vi "Insert Subroutine.vi"(8 "error in (no error)":errorcluster, 10 "Insert Subroutine":T1, 11 "Test Executive Builder in":refnum<class "Test Executive Builder.lvclass">) -> (0 "error out":errorcluster, 3 "Test Executive Builder out":refnum<class "Test Executive Builder.lvclass">, 5 "Unique ID out":string)   [LabVIEW 2017, in "Test Executive Builder.lvclass"]
uses:
  Test Executive Builder.lvclass
  Source/Test Executive Builder Model/Test Executive Builder Model/Test Executive Builder Model.lvclass
  e5ad1a27-23be-4da1-be5e-5f15b9041f0f.vi
  <vilib>/gpm_packages/@cs/mva-core/Source/IModel/IModel/IModel.lvclass
  C:/Users/jonmc/Documents/Git/Test Executive Builder/Source/Test Executive Builder Model/Test Executive Builder Model/Test Executive Builder Model.lvclass
  C:/Users/jonmc/Documents/Git/Test Executive Builder/gpm_packages/@cs/mva-core/Source/IModel/IModel/IModel.lvclass
  Source/Test Executive Builder Dialogs/ITest Executive Builder Dialog/ITest Executive Builder Dialog.lvclass
  Source/Application Dependencies/Insert Subroutine.ctl
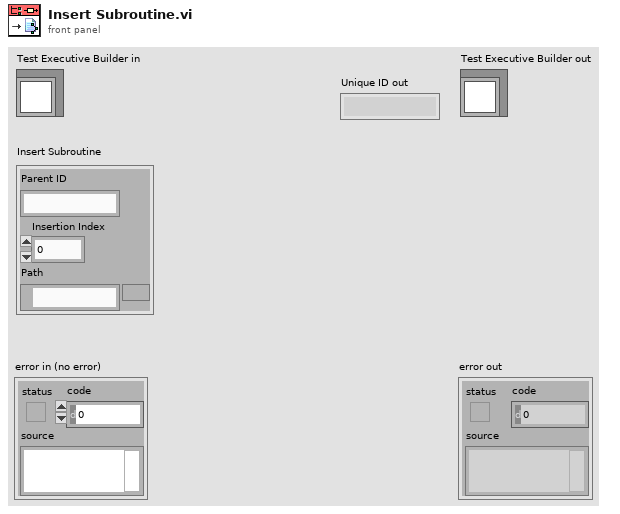
[diagram p1: front panel]
types:
  T1 = typedef "Insert Subroutine.ctl" = cluster{"Parent ID":string, "Insertion Index":i32, "Path":path}
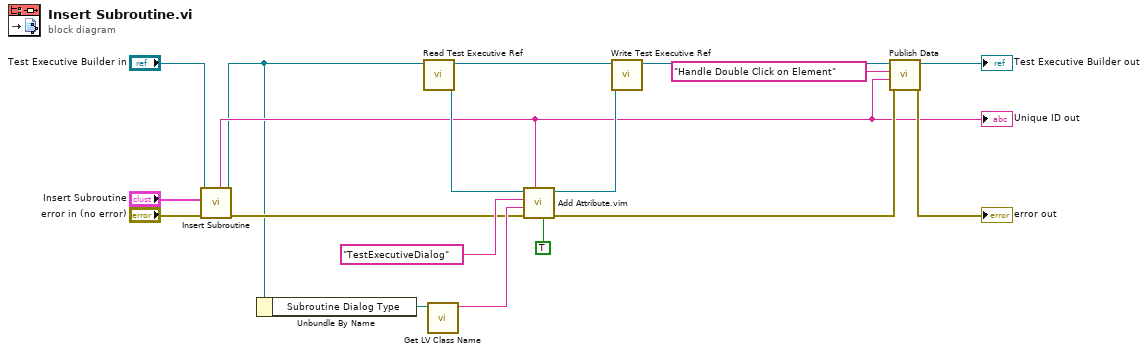
[diagram p0: block diagram]
diagram:
  n1 = call-parent "Insert Subroutine.vi"("error in (no error)"="error in (no error)", "Insert Subroutine"="Insert Subroutine", "Test Executive Builder Model in"="Test Executive Builder in") -> ("error out"=w5:errorcluster, "Test Executive Builder Model out"=w2:refnum<class "Test Executive Builder.lvclass">, "Unique ID out"=w3:string)  [unwired: 6 in]
  "Unique ID out" <- w3
  n2 = Unbundle By Name(w2) -> ("Subroutine Dialog Type"=w1:refnum<class "ITest Executive Builder Dialog.lvclass">)
  n3 = call "Read Test Executive Ref.vi"("Test Executive Builder Model in"=w2) -> ("Test Executive Ref"=w14:refnum<data-value>, "Test Executive Builder Model out"=w15:refnum<class "Test Executive Builder.lvclass">)  [unwired: 9 in]
  n4 = call <vilib>:"Get LV Class Name.vi"("object"=w1) -> ("class name"=w10:string)  [unwired: 9 in, 1 out]
  n5 = call "Add Attribute.vim"("Private?"=TRUE, "ID"=w3, "error in (no error)"=w5, "Attribute"=w10, "Attribute Name"="TestExecutiveDialog", "Test Executive Ref"=w14) -> ("error out"=w7:errorcluster, "Test Executive Ref out"=w13:refnum<data-value>)  [unwired: 2 in, 2 out]
  n6 = call "Write Test Executive Ref.vi"("Test Executive Ref"=w13, "Test Executive Builder Model in"=w15) -> ("Test Executive Builder Model out"=w8:refnum<class "Test Executive Builder.lvclass">)  [unwired: 9 in]
  n7 = call <vilib>:"Publish Data.vi"("error in (no error)"=w7, "Data to Publish"=w3, "Datum Name"="Handle Double Click on Element", "IModel in"=w8) -> ("error out"=→"error out":errorcluster, "IModel out"=→"Test Executive Builder out":refnum<class "Test Executive Builder.lvclass">)  [unwired: 6 in]
